vi "check_variant.vi"(10 "String":string="0123456789.+-") -> (0 "contains decimal":bool, 1 "string portion":string, 2 "contains non-numeric":bool)   [LabVIEW 2024, in "CLZ_to_ComicVine.lvlib"]
uses:
  CLZ_to_ComicVine.lvlib
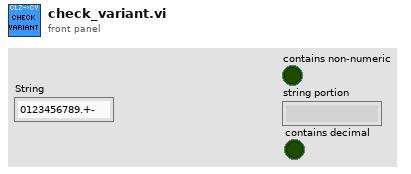
[diagram p1: front panel]
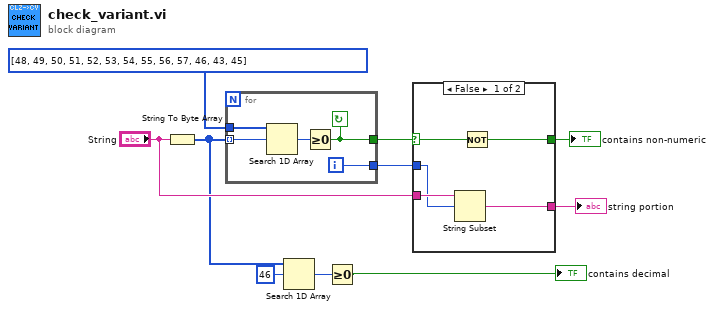
[diagram p0: block diagram]
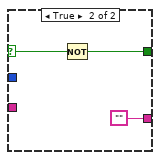
[diagram p2: hidden frame]
diagram:
  n1 = String To Byte Array(string="String") -> (unsigned byte array=w4:u8[])
  n2 = for {
    tunnel: w4 -> [w14] mode=indexing
    tunnel: u8[] [48, 49, 50, 51, 52, 53, 54, 55, 56, 57, 46, 43, 45] ("unsigned byte array 2") -> [w15]
    tunnel: [w11] -> w5
    tunnel: [w12] -> w9
    i -> [w11]
    stop <- w12 continue-if-true
    n3 = Search 1D Array(1D array=w15, element=w14) -> (index of element=w13:i32)  [unwired: 1 in]
    n4 = Greater Or Equal To 0?(x=w13) -> (x >= 0?=w12:bool)
  }
  n5 = Search 1D Array(1D array=w4, element=u8 46) -> (index of element=w2:i32)  [unwired: 1 in]
  n6 = Greater Or Equal To 0?(x=w2) -> (x >= 0?=→"contains decimal":bool)
  n7 = case shown="False" w9 {
    selector: w9 -> [w20 w22]
    tunnel: w5 -> [w16 _]
    tunnel: [w18 ""] -> w7
    tunnel: [w19 w21] -> w8
    tunnel: "String" -> [w17 _]
    frame False {
      n8 = String Subset(string=w17, offset (0)=w16) -> (substring=w18:string)  [unwired: 1 in]
      n9 = Not(x=w20) -> (.not. x?=w19:bool)
    }
    frame True {
      n10 = Not(x=w22) -> (.not. x?=w21:bool)
    }
  }
  "contains non-numeric" <- w8
  "string portion" <- w7
